vi "Chemical Dissolution Chamber.vi"(5 "Gas Upgrades":u32 max=8, 7 "Speed Upgrades":u32 max=8, 11 "Sulfuric Acid (mB/t)":ext) -> (0 "Input Limiting":bool, 1 "Limiting":bool, 2 "Required Items/t":ext, 3 "Hydrofluoric Acid (mB/t)":u32, 4 "Required Items/s":ext, 6 "Gas Required (mB/t)":ext)   [LabVIEW 2023]
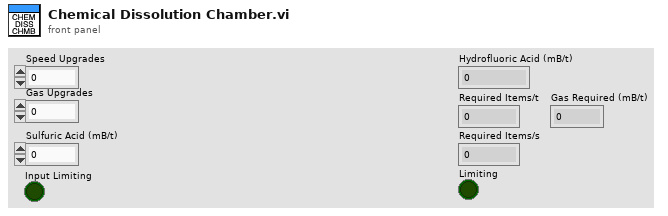
[diagram p1: front panel]
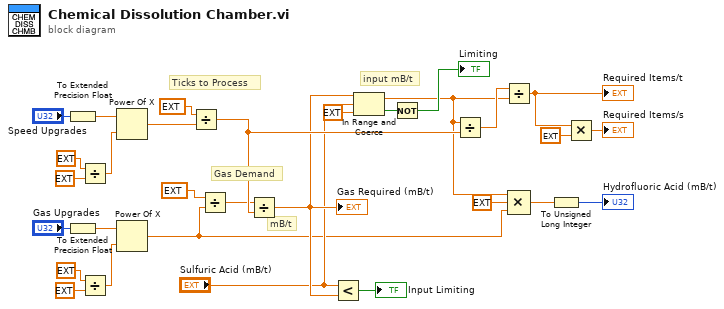
[diagram p0: block diagram]
diagram:
  # "input mB/t"
  # "mB/t"
  # "Gas Demand"
  # "Ticks to Process"
  n1 = To Extended Precision Float(1:"Speed Upgrades") -> (0:w21:ext)
  n2 = To Extended Precision Float(1:"Gas Upgrades") -> (0:w8:ext)
  n3 = Divide(x=ext 4.0, y=ext 3.0) -> (x/y=w25:ext)
  n4 = Divide(x=ext 4.0, y=ext 3.0) -> (x/y=w7:ext)
  n5 = Power Of X(1:w25, 2:w21) -> (0:w29:ext)
  n6 = Power Of X(1:w7, 2:w8) -> (0:w1:ext)
  n7 = Divide(x=ext 100.0 ("y"), y=w29) -> (x/y=w16:ext)
  n8 = Divide(x=ext 100.0, y=w1) -> (x/y=w2:ext)
  n9 = Divide(x=w2, y=w16) -> (x/y=w15:ext)
  "Gas Required (mB/t)" <- w15
  n10 = Less?(x="Sulfuric Acid (mB/t)", y=w15) -> (x < y?=→"Input Limiting":bool)
  n11 = In Range and Coerce(upper limit=w15, x="Sulfuric Acid (mB/t)", lower limit=ext 0.0) -> (coerced(x)=w13:ext, In Range?=w18:bool)
  n12 = Not(x=w18) -> (.not. x?=→"Limiting":bool)
  n13 = Divide(x=w13, y=w16) -> (x/y=w14:ext)
  n14 = Divide(x=w14, y=w13) -> (x/y=w22:ext)
  "Required Items/t" <- w22
  n15 = Compound Arithmetic op=MULTIPLY(w13, ext 10.0 ("y"), w1) -> (w10:ext)
  n16 = To Unsigned Long Integer(number=w10) -> (unsigned 32bit integer=→"Hydrofluoric Acid (mB/t)":u32)
  n17 = Multiply(x=w22, y=ext 20.0) -> (x*y=→"Required Items/s":ext)
